vi "Send State Message from Inspection StateMachine_MI.vi"(7 "Message Priority (Normal)":T1=enum."Normal", 8 "error in (no error)":errorcluster, 10 "State Message from Inspection Statemachine":string, 11 "Message Enqueuer":refnum<class "Message Enqueuer.lvclass">) -> (0 "error out":errorcluster, 3 "Message Enqueuer out":refnum<class "Message Enqueuer.lvclass">)   [LabVIEW 2015, in "State Message from Inspection StateMachine Msg_MI.lvclass"]
doc: "This VI sends the message to an actor."
uses:
  State Message from Inspection StateMachine Msg_MI.lvclass
  <vilib>/ActorFramework/Message Enqueuer/Message Enqueuer.lvclass
  <vilib>/ActorFramework/Message Enqueuer/Message Priority.ctl
  State Message from Inspection StateMachine Msg_MI.lvclass/State Message from Inspection StateMachine Msg_MI.ctl
  <vilib>/ActorFramework/Message Enqueuer/Message Enqueuer.lvclass/Message Enqueuer.ctl
  <vilib>/ActorFramework/Message Priority Queue/Priority Enqueue.vi
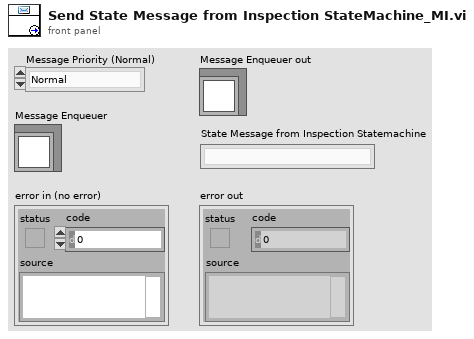
[diagram p1: front panel]
types:
  T1 = typedef "Actor Framework.lvlib/Message Enqueuer.lvclass/Message Priority.ctl" = enum16{"Low", "Normal", "High"}
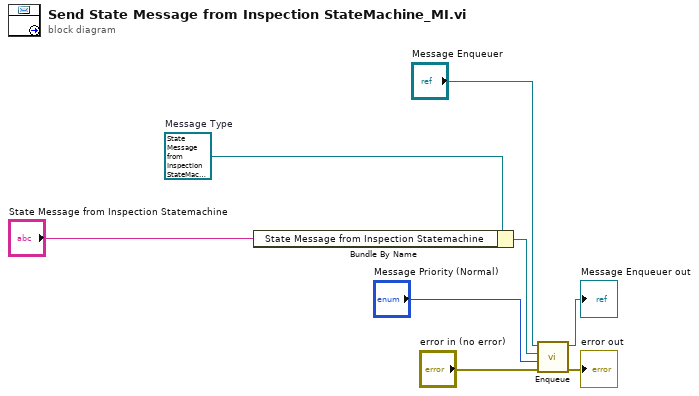
[diagram p0: block diagram]
diagram:
  w3 = refnum<class "State Message from Inspection StateMachine Msg_MI.lvclass"> refnum  # Message Type
  n1 = Bundle By Name(cluster=w3, "State Message from Inspection Statemachine"="State Message from Inspection Statemachine") -> (w2:refnum<class "State Message from Inspection StateMachine Msg_MI.lvclass">)
  n2 = call <vilib>:"Enqueue.vi"("error in (no error)"="error in (no error)", "Message Priority (Normal)"="Message Priority (Normal)", "Message"=w2, "Message Enqueuer in"="Message Enqueuer") -> ("error out"=→"error out":errorcluster, "Message Enqueuer out"=→"Message Enqueuer out":refnum<class "Message Enqueuer.lvclass">)  [unwired: 6 in]
